vi "IMPRIMER ETIQUETTE EMBALLAGE AVEC SCAN.vi"() -> ()   [LabVIEW 2011]
panel:
  in  "Nb total de valves":string="100"
  in  "indice client":string="03"
  in  "N°article client":string="EL-360 "
  in  "Société de facturation":string(combo)="Fluid Automation Systems SA"
  in  "Affiche code bar client":string(combo)="OUI"
  in  "n° commande FAS":string="03838/08-07.01.01"
  out "n° valves 11-15":string
  out "Ref client":string="EL-360 "
  in  "Langue":string(combo)="E"
  out "nom sous code bar client":string="EL-360  03 08010802 7"
  out "n° valves 46-50":string
  out "n° valves 41-45":string
  out "n° valves 36-40":string
  in  "destinataire":string="Saime"
  in  "n° cmde client":string="CF-08-0253/2"
  out "n° valves 31-35":string
  out "n° valves 26-30":string
  out "n° valves 21-25":string
  out "n° valves 16-20":string
  out "n° valves 6-10":string="08020006, 08020066"
  out "n° valves 1-5":string="08010003, 08010006, 08010009, 08010022, 08010099"
  out "Quantité":string="7/100"
  in  "carton":string="1/1"
  in  "nom valve FAS":string="12-216C-04520 EQIFIL 104mA 36ohm"
  out "chaine  à écrire":string="ZB\nUS\nq600\nD7\nN\nR150,20\nI8,12,001\rA0,40,0,2,1,1,N,\"Carton : 1/2\"\rA0,85,0,2,1,1,N,\"Nb de valves : 25\"\rA0,130,0,2,1,1,N,\"Nø valves :\"\rA144,130,0,1,1,1,N,\"04235698, 05050505, 06060606, 06125478\"\rA144,146,0,1,1,1,N,\"06235511, 07070707, 08023326, 08080808\"\rA144,162,0,1,1,1,N,\"08080808, 08090909, 08110030, 08112347\"\rA144,178,0,1,1,1,N,\"08120003, 08120004, 08120025, 08121114\"\rA144,194,0,1,1,1,N,\"08123625, 08141254, 08152365, 08235644\"\rA144,210,0,1,1,1,N,\"08336251, 08452145, 08521456, 09040006\"\rA144,226,0,1,1,1,N,\"09090909\"\rB64,260,0,1,1,20,56,N,\"12-216C-04520 EQIFIL 104mA 36ohm\"\rA58,324,0,3,1,1,N,\"12..."
  in  "Tableau n° valves":string[](array[string])=["08010022", "08010003", "08020006", "08010006", "08010009", "08020066", "08010099"]
  # "Destinataire:"
  # "N°commande :"
  # "Carton :"
  # "Quantité:"
  # "Votre ref.:"
  # "N° valves :\n(P/N)"
  # "FASmedic s.a.\nZone industrielle\nCH-1607 Palézieux-Gare\nTél.+41(0)21 907 79 71\nwww.fasmedic.com"
  # "N°article FAS:"
  # "N°commande FAS:"
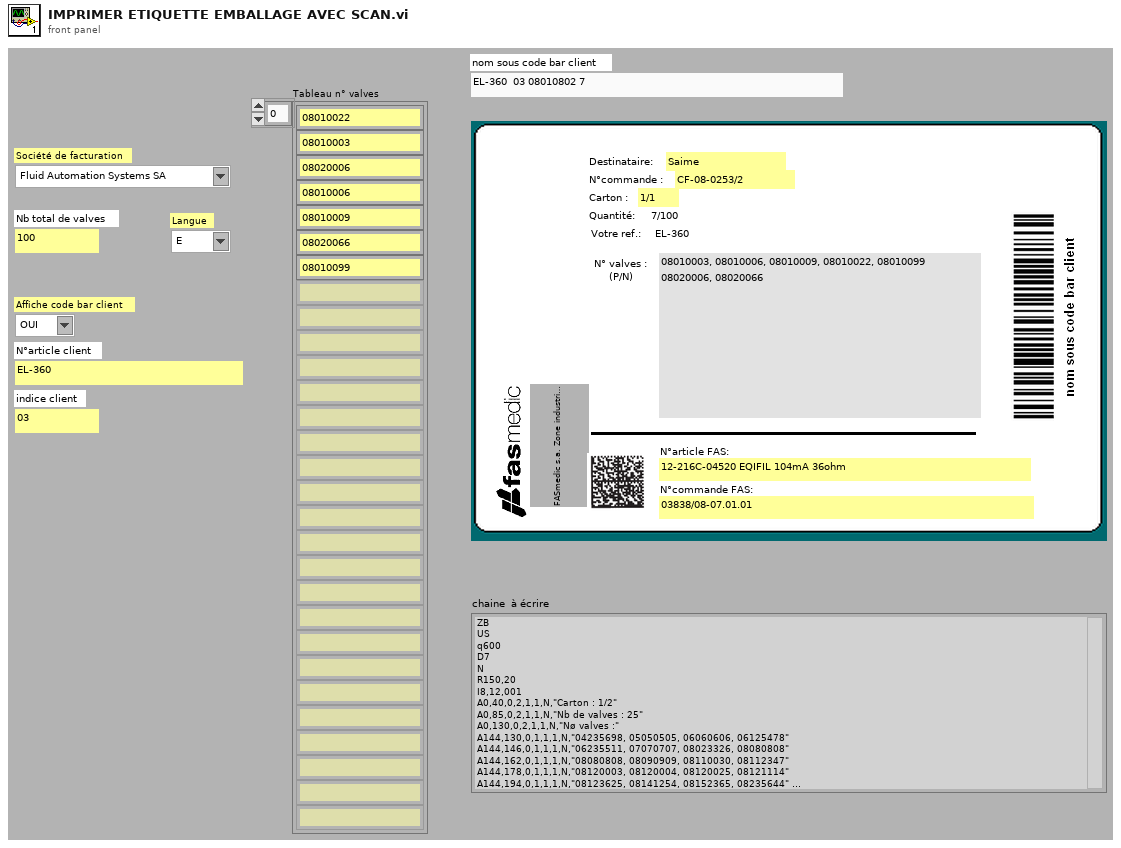
[diagram p1: front panel]
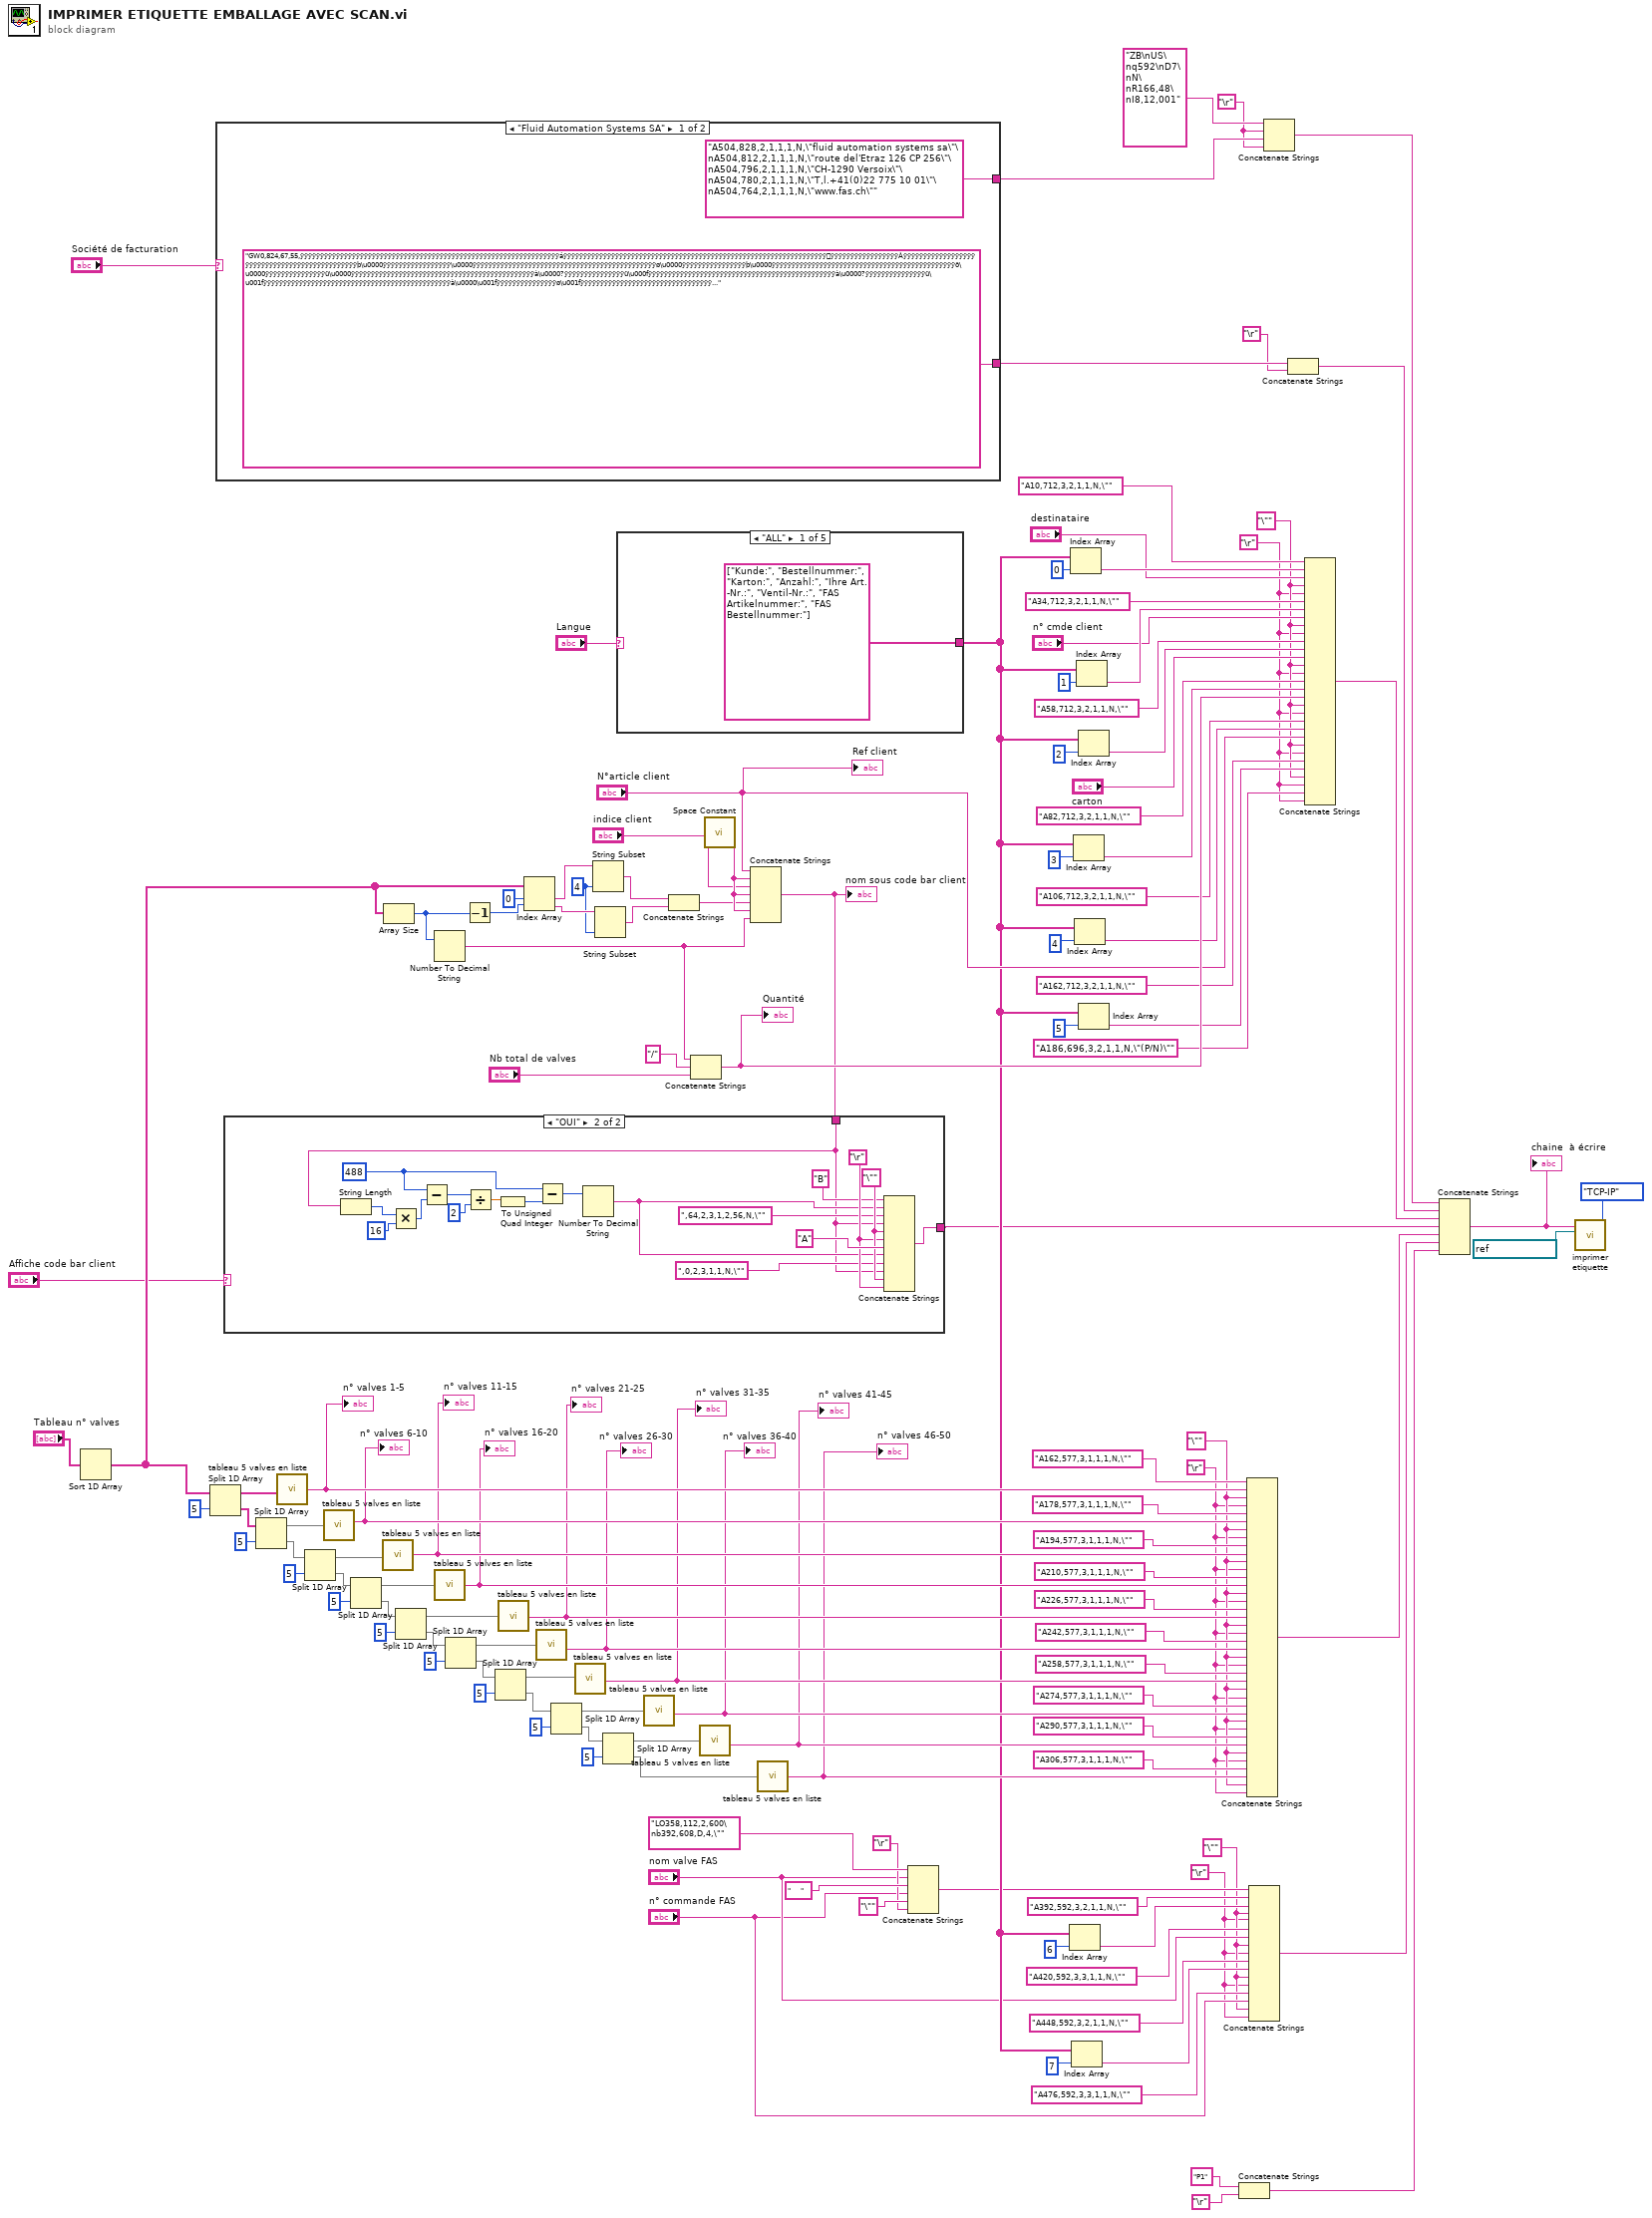
[diagram p0: block diagram]
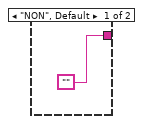
[diagram p2: hidden frame]
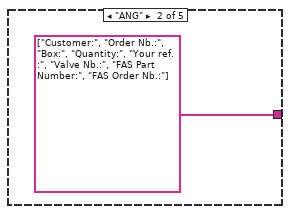
[diagram p3: hidden frame]
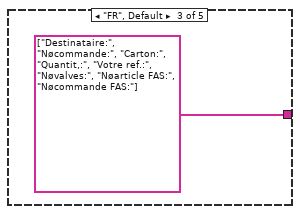
[diagram p4: hidden frame]
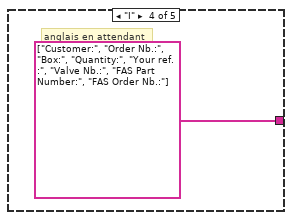
[diagram p5: hidden frame]
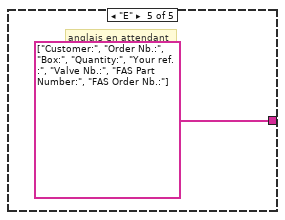
[diagram p6: hidden frame]
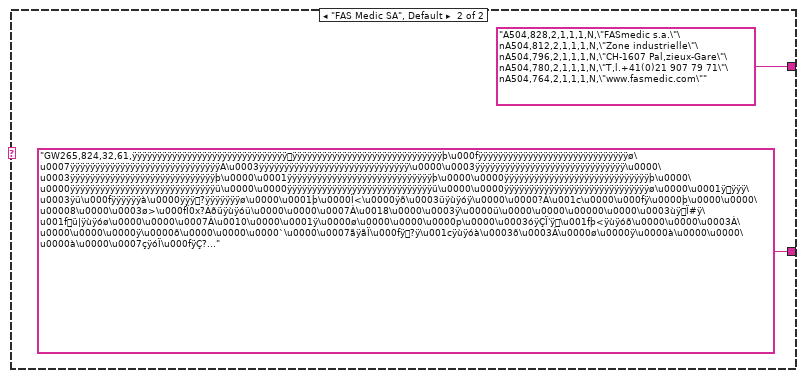
[diagram p7: hidden frame]
diagram:
  w17 = "\r"
  w18 = "\""
  w36 = "\""
  w35 = "\r"
  w59 = "\""
  w57 = "\r"
  w83 = "\r"
  w97 = 4 ("longueur (reste)")
  n1 = Sort 1D Array(array="Tableau n° valves") -> (sorted array=w92:string[])
  n2 = Split 1D Array(array=w92, index=5 ("indice")) -> (first subarray=w121:string[], second subarray=w128:string[])
  n3 = case shown="\"Fluid Automation Systems SA\"" "Société de facturation" {
    tunnel: ["GW0,824,67,55,ÿÿÿÿÿÿÿÿÿÿÿÿÿÿÿÿÿÿÿÿÿÿÿÿÿÿÿÿÿÿÿÿÿÿÿÿÿÿÿÿÿÿÿÿÿÿÿÿÿÿÿÿÿÿÿÿÿÿÿÿÿÿÿÿÿáÿÿÿÿÿÿÿÿÿÿÿÿÿÿÿÿÿÿÿÿÿÿÿÿÿÿÿÿÿÿÿÿÿÿÿÿÿÿÿÿÿÿÿÿÿÿÿÿÿÿÿÿÿÿÿÿÿÿÿÿÿÿÿÿÿÿÿÿÿÿÿÿÿÿÿÿÿÿÿÿÿÿÿÀÿÿÿÿÿÿÿÿÿÿÿÿÿÿÿÿÿÿÿÿÿÿÿÿÿÿÿÿÿÿÿÿÿÿÿÿÿÿÿÿÿÿÿÿÿÿþ\u0000ÿÿÿÿÿÿÿÿÿÿÿÿÿÿÿÿÿ\u0000ÿÿÿÿÿÿÿÿÿÿÿÿÿÿÿÿÿÿÿÿÿÿÿÿÿÿÿÿÿÿÿÿÿÿÿÿÿÿÿÿÿÿÿÿÿÿø\u0000ÿÿÿÿÿÿÿÿÿÿÿÿÿÿÿÿþ\u0000ÿÿÿÿÿÿÿÿÿÿÿÿÿÿÿÿÿÿÿÿÿÿÿÿÿÿÿÿÿÿÿÿÿÿÿÿÿÿÿÿÿÿÿÿÿÿð\u0000ÿÿÿÿÿÿÿÿÿÿÿÿÿÿÿü\u0000ÿÿÿÿÿÿÿÿÿÿÿÿÿÿÿÿÿÿÿÿÿÿÿÿÿÿÿÿÿÿÿÿÿÿÿÿÿÿÿÿÿÿÿÿÿÿà\u0000?ÿÿÿÿÿÿÿÿÿÿÿÿÿÿÿü\u000fÿÿÿÿÿÿÿÿÿÿÿÿÿÿÿÿÿÿÿÿÿÿÿÿÿÿÿÿÿÿÿÿÿÿÿÿÿÿÿÿÿÿÿÿÿÿÿà\u0000?ÿÿÿÿÿÿÿÿÿÿÿÿÿÿÿü\u001fÿÿÿÿÿÿÿÿÿÿÿÿÿÿÿÿÿÿÿÿÿÿÿÿÿÿÿÿÿÿÿÿÿÿÿÿÿÿÿÿÿÿÿÿÿÿÿà\u0000\u001fÿÿÿÿÿÿÿÿÿÿÿÿÿÿÿø\u001fÿÿÿÿÿÿÿÿÿÿÿÿÿÿÿÿÿÿÿÿÿÿÿÿÿÿÿÿÿÿÿÿÿ..." "GW265,824,32,61,ÿÿÿÿÿÿÿÿÿÿÿÿÿÿÿÿÿÿÿÿÿÿÿÿÿÿÿÿÿÿÿÿÿÿÿÿÿÿÿÿÿÿÿÿÿÿÿÿÿÿÿÿÿÿÿÿÿÿÿÿÿþ\u000fÿÿÿÿÿÿÿÿÿÿÿÿÿÿÿÿÿÿÿÿÿÿÿÿÿÿÿÿÿÿø\u0007ÿÿÿÿÿÿÿÿÿÿÿÿÿÿÿÿÿÿÿÿÿÿÿÿÿÿÿÿÿÿÀ\u0003ÿÿÿÿÿÿÿÿÿÿÿÿÿÿÿÿÿÿÿÿÿÿÿÿÿÿÿÿÿÿ\u0000\u0003ÿÿÿÿÿÿÿÿÿÿÿÿÿÿÿÿÿÿÿÿÿÿÿÿÿÿÿÿÿÿ\u0000\u0003ÿÿÿÿÿÿÿÿÿÿÿÿÿÿÿÿÿÿÿÿÿÿÿÿÿÿÿÿÿþ\u0000\u0001ÿÿÿÿÿÿÿÿÿÿÿÿÿÿÿÿÿÿÿÿÿÿÿÿÿÿÿÿÿþ\u0000\u0000ÿÿÿÿÿÿÿÿÿÿÿÿÿÿÿÿÿÿÿÿÿÿÿÿÿÿÿÿÿþ\u0000\u0000ÿÿÿÿÿÿÿÿÿÿÿÿÿÿÿÿÿÿÿÿÿÿÿÿÿÿÿÿÿü\u0000\u0000ÿÿÿÿÿÿÿÿÿÿÿÿÿÿÿÿÿÿÿÿÿÿÿÿÿÿÿÿÿü\u0000\u0000ÿÿÿÿÿÿÿÿÿÿÿÿÿÿÿÿÿÿÿÿÿÿÿÿÿÿÿÿÿø\u0000\u0001ÿÿÿÿ\u0003ÿü\u000fÿÿÿÿÿÿà\u0000ÿÿÿ?ÿÿÿÿÿÿÿø\u0000\u0001þ\u0000Ï<\u0000ÿð\u0003üÿùÿóÿ\u0000\u0000?À\u001c\u0000\u000fÿ\u0000þ\u0000\u0000\u00008\u0000\u0003ø>\u000fÏ0x?Áðüÿùÿóü\u0000\u0000\u0007À\u0018\u0000\u0003ÿ\u0000ü\u0000\u0000\u00000\u0000\u0003ùÿÏ#ÿ\u001fü|ÿùÿóø\u0000\u0000\u0007À\u0010\u0000\u0001ÿ\u0000ø\u0000\u0000\u0000p\u0000\u0003óÿÇÏ'ÿ\u001fþ<ÿùÿóð\u0000\u0000\u0003À\u0000\u0000\u0000ÿ\u0000ð\u0000\u0000\u0000`\u0000\u0007ãÿãÏ\u000fÿ?ÿ\u001cÿùÿóà\u0003ð\u0003À\u0000ø\u0000ÿ\u0000à\u0000\u0000\u0000à\u0000\u0007çÿóÏ\u000fÿÇ?..."] -> w14
    tunnel: ["A504,828,2,1,1,1,N,\"fluid automation systems sa\"\nA504,812,2,1,1,1,N,\"route del'Etraz 126 CP 256\"\nA504,796,2,1,1,1,N,\"CH-1290 Versoix\"\nA504,780,2,1,1,1,N,\"T‚l.+41(0)22 775 10 01\"\nA504,764,2,1,1,1,N,\"www.fas.ch\"" "A504,828,2,1,1,1,N,\"FASmedic s.a.\"\nA504,812,2,1,1,1,N,\"Zone industrielle\"\nA504,796,2,1,1,1,N,\"CH-1607 Pal‚zieux-Gare\"\nA504,780,2,1,1,1,N,\"T‚l.+41(0)21 907 79 71\"\nA504,764,2,1,1,1,N,\"www.fasmedic.com\""] -> w84
    frame "Fluid Automation Systems SA" {
    }
    frame "FAS Medic SA", Default {
    }
  }
  n4 = Split 1D Array(array=w128, index=5 ("indice")) -> (first subarray=w120:string[], second subarray=w126:string[])
  n5 = call "tableau 5 valves en liste.vi"("Tableau de 5 valves"=w121) -> ("Chaîne de 5 valves"=w55:string)
  "n° valves 1-5" <- w55
  n6 = Split 1D Array(array=w126, index=5 ("indice")) -> (first subarray=w119:string[], second subarray=w124:string[])
  n7 = call "tableau 5 valves en liste.vi"("Tableau de 5 valves"=w120) -> ("Chaîne de 5 valves"=w53:string)
  "n° valves 6-10" <- w53
  n8 = Split 1D Array(array=w124, index=5 ("indice")) -> (first subarray=w118:string[], second subarray=w122:string[])
  n9 = call "tableau 5 valves en liste.vi"("Tableau de 5 valves"=w119) -> ("Chaîne de 5 valves"=w52:string)
  "n° valves 11-15" <- w52
  n10 = Array Size(array=w92) -> (size(s)=w91:i32)
  n11 = Split 1D Array(array=w122, index=5 ("indice")) -> (first subarray=w117:string[], second subarray=w115:string[])
  n12 = Number To Decimal String(number=w91) -> (decimal integer string=w87:string)  [unwired: 1 in]
  n13 = call "tableau 5 valves en liste.vi"("Tableau de 5 valves"=w118) -> ("Chaîne de 5 valves"=w49:string)
  "n° valves 16-20" <- w49
  n14 = Split 1D Array(array=w115, index=5 ("indice")) -> (first subarray=w114:string[], second subarray=w112:string[])
  n15 = Decrement(x=w91) -> (x-1=w94:i32)
  n16 = Split 1D Array(array=w112, index=5 ("indice")) -> (first subarray=w111:string[], second subarray=w109:string[])
  n17 = call "tableau 5 valves en liste.vi"("Tableau de 5 valves"=w117) -> ("Chaîne de 5 valves"=w48:string)
  "n° valves 21-25" <- w48
  n18 = Index Array(array=w92, index #1=0 ("indice"), index #2=w94) -> (element #1=w99:string, element #2=w98:string)
  n19 = call "tableau 5 valves en liste.vi"("Tableau de 5 valves"=w114) -> ("Chaîne de 5 valves"=w45:string)
  "n° valves 26-30" <- w45
  n20 = Split 1D Array(array=w109, index=5 ("indice")) -> (first subarray=w108:string[], second subarray=w106:string[])
  n21 = call "tableau 5 valves en liste.vi"("Tableau de 5 valves"=w111) -> ("Chaîne de 5 valves"=w43:string)
  "n° valves 31-35" <- w43
  n22 = String Subset(string=w99, length (rest)=w97) -> (substring=w96:string)  [unwired: 1 in]
  n23 = String Subset(string=w98, length (rest)=w97) -> (substring=w95:string)  [unwired: 1 in]
  n24 = Split 1D Array(array=w106, index=5 ("indice")) -> (first subarray=w105:string[], second subarray=w104:string[])
  n25 = case shown="\"ALL\"" "Langue" {
    tunnel: [string[] ["Kunde:", "Bestellnummer:", "Karton:", "Anzahl:", "Ihre Art.-Nr.:", "Ventil-Nr.:", "FAS Artikelnummer:", "FAS Bestellnummer:"] string[] ["Customer:", "Order Nb.:", "Box:", "Quantity:", "Your ref.:", "Valve Nb.:", "FAS Part Number:", "FAS Order Nb.:"] string[] ["Destinataire:", "Nøcommande:", "Carton:", "Quantit‚:", "Votre ref.:", "Nøvalves:", "Nøarticle FAS:", "Nøcommande FAS:"] string[] ["Customer:", "Order Nb.:", "Box:", "Quantity:", "Your ref.:", "Valve Nb.:", "FAS Part Number:", "FAS Order Nb.:"] string[] ["Customer:", "Order Nb.:", "Box:", "Quantity:", "Your ref.:", "Valve Nb.:", "FAS Part Number:", "FAS Order Nb.:"]] -> w29
    frame "ALL" {
    }
    frame "ANG" {
    }
    frame "FR", Default {
    }
    frame "I" {
      # "anglais en attendant"
    }
    frame "E" {
      # "anglais en attendant"
    }
  }
  n26 = call "tableau 5 valves en liste.vi"("Tableau de 5 valves"=w108) -> ("Chaîne de 5 valves"=w41:string)
  "n° valves 36-40" <- w41
  n27 = Concatenate Strings(w96, w95) -> (w100:string)
  n28 = Concatenate Strings(w87, "/" ("chaîne"), "Nb total de valves") -> (w67:string)
  "Quantité" <- w67
  n29 = call "tableau 5 valves en liste.vi"("Tableau de 5 valves"=w105) -> ("Chaîne de 5 valves"=w39:string)
  "n° valves 41-45" <- w39
  n30 = call <vilib>:"Space Constant.vi"() -> ("String"=w101:string)
  n31 = Concatenate Strings("N°article client", w101, "indice client", w101, w100, w101, w87) -> (w5:string)
  "nom sous code bar client" <- w5
  n32 = case shown="\"OUI\"" "Affiche code bar client" {
    tunnel: w5 -> [_ w141]
    tunnel: ["" w155] -> w4
    frame "NON", Default {
    }
    frame "OUI" {
      w149 = 488
      w157 = "\""
      w156 = "\r"
      n33 = String Length(string=w141) -> (length=w154:i32)
      n34 = Multiply(x=w154, y=16) -> (x*y=w152:i32)
      n35 = Subtract(x=w149, y=w152) -> (x-y=w151:i32)
      n36 = Divide(x=w151, y=2) -> (x/y=w148:dbl)
      n37 = To Unsigned Quad Integer(1:w148) -> (0:w147:u64)
      n38 = Subtract(x=w149, y=w147) -> (x-y=w146:u64)
      n39 = Number To Decimal String(number=w146) -> (decimal integer string=w142:string)  [unwired: 1 in]
      n40 = Concatenate Strings("B", w142, ",64,2,3,1,2,56,N,\"", w141, w157, w156, "A", w142, ",0,2,3,1,1,N,\"", w141, w157, w156) -> (w155:string)
    }
  }
  n41 = call "tableau 5 valves en liste.vi"("Tableau de 5 valves"=w104) -> ("Chaîne de 5 valves"=w37:string)
  "n° valves 46-50" <- w37
  n42 = Concatenate Strings("LO358,112,2,600\nb392,608,D,4,\"", "nom valve FAS", "     ", "n° commande FAS", "\"", "\r") -> (w27:string)
  n43 = Index Array(array=w29, index=6 ("indice")) -> (element=w25:string)
  n44 = Index Array(array=w29, index=0 ("indice")) -> (element=w80:string)
  n45 = Index Array(array=w29, index=7 ("indice")) -> (element=w21:string)
  n46 = Index Array(array=w29, index=3 ("indice")) -> (element=w68:string)
  n47 = Index Array(array=w29, index=4 ("indice")) -> (element=w65:string)
  n48 = Index Array(array=w29, index=1 ("indice")) -> (element=w76:string)
  n49 = Index Array(array=w29, index=2 ("indice")) -> (element=w72:string)
  n50 = Index Array(array=w29, index=5 ("indice")) -> (element=w60:string)
  n51 = Concatenate Strings("P1", "\r") -> (w7:string)
  n52 = Concatenate Strings("A162,577,3,1,1,1,N,\"", w55, w36, w35, "A178,577,3,1,1,1,N,\"", w53, w36, w35, "A194,577,3,1,1,1,N,\"", w52, w36, w35, "A210,577,3,1,1,1,N,\"", w49, w36, w35, "A226,577,3,1,1,1,N,\"", w48, w36, w35, "A242,577,3,1,1,1,N,\"", w45, w36, w35, "A258,577,3,1,1,1,N,\"", w43, w36, w35, "A274,577,3,1,1,1,N,\"", w41, w36, w35, "A290,577,3,1,1,1,N,\"", w39, w36, w35, "A306,577,3,1,1,1,N,\"", w37, w36, w35) -> (w9:string)
  n53 = Concatenate Strings(w27, "A392,592,3,2,1,1,N,\"", w25, w18, w17, "A420,592,3,3,1,1,N,\"", "nom valve FAS", w18, w17, "A448,592,3,2,1,1,N,\"", w21, w18, w17, "A476,592,3,3,1,1,N,\"", "n° commande FAS", w18, w17) -> (w8:string)
  n54 = Concatenate Strings("ZB\nUS\nq592\nD7\nN\nR166,48\nI8,12,001", w83, w84, w83) -> (w12:string)
  n55 = Concatenate Strings(w14, "\r") -> (w11:string)
  n56 = Concatenate Strings("A10,712,3,2,1,1,N,\"", w80, "destinataire", w59, w57, "A34,712,3,2,1,1,N,\"", w76, "n° cmde client", w59, w57, "A58,712,3,2,1,1,N,\"", w72, "carton", w59, w57, "A82,712,3,2,1,1,N,\"", w68, w67, w59, w57, "A106,712,3,2,1,1,N,\"", w65, "N°article client", w59, w57, "A162,712,3,2,1,1,N,\"", w60, w59, w57, "A186,696,3,2,1,1,N,\"(P/N)\"", w57) -> (w10:string)
  n57 = Concatenate Strings(w12, w11, w10, w4, w9, w8, w7) -> (w6:string)
  "chaine  à écrire" <- w6
  n58 = call "imprimer etiquette.vi"("Type de liaison"=enum16{"RS232", "USB", "TCP-IP", "Aucune"}."TCP-IP", "Nom de ressource VISA TCP-IP"=refnum<visa-resource-name> "TLP3844-Z", "chaine à écrire"=w6) -> ()  [unwired: 7 in, 1 out]
  "Ref client" <- "N°article client"
